vi "Init Msg Default.vi"() -> (3 "Stopping Msg out":refnum<class "Stopping Msg.lvclass">)   [LabVIEW 2020, in "jettl.lvlib" / "Stopping jettl Msg.lvlib" / "Stopping Msg.lvlib" / "Stopping Msg.lvclass"]
doc: "jettl 6.12.1.94\nNathan Davis - Nathan Davis\nCopyright (c) 2026, Nathan Davis\nMIT"
uses:
  Stopping Msg.lvclass
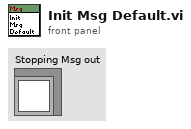
[diagram p1: front panel]
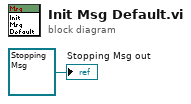
[diagram p0: block diagram]
diagram:
  "Stopping Msg out" <- refnum<class "Stopping Msg.lvclass"> refnum ("TEMPLATE Msg out")
